vi "UART_With_Buffer.vi"(0 "COM":refnum<visa-resource-name>, 1 "Send":string(combo), 3 "Timeout (ms)":u32=500, 5 "Function":T1(ring)=enum."SendWaitRead", 9 "Baudrate":u32=3000000, 11 "error in (no error)":errorcluster, 12 "REC":string) -> (4 "ReceiveString":string, 6 "pass?":bool, 10 "Return":string, 15 "error out":errorcluster)   [LabVIEW 2020, in "UART.lvlib"]
uses:
  UART.lvlib
  <vilib>/Instr/_visa.llb/VISA Set IO Buffer Mask.ctl
  <vilib>/Instr/_visa.llb/VISA Flush IO Buffer Mask.ctl
  4a145ab3-8364-4eaa-b6a3-0a612f5f0f50.vi
  75df8ced-9b69-4a5e-8517-458ef4cbff5d.vi
  <vilib>/Instr/_visa.llb/VISA Configure Serial Port (Instr).vi
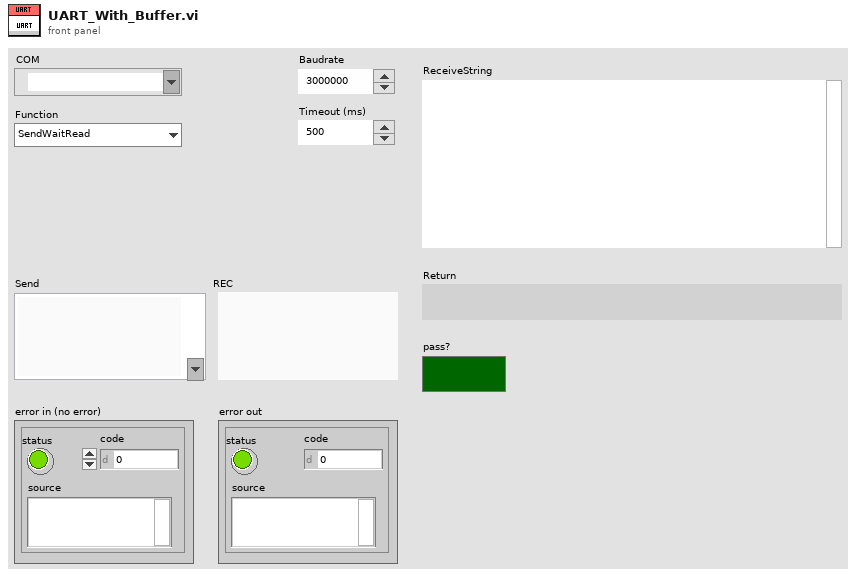
[diagram p1: front panel]
types:
  T1 = enum16{"Open", "Close", "ClearBuffer", "Send", "Read", "SendWaitRead", "SendCompare", "ReadCompare"}
  T2 = typedef "VISA Set IO Buffer Mask.ctl" = u16
  T3 = typedef "VISA Flush IO Buffer Mask.ctl" = u16
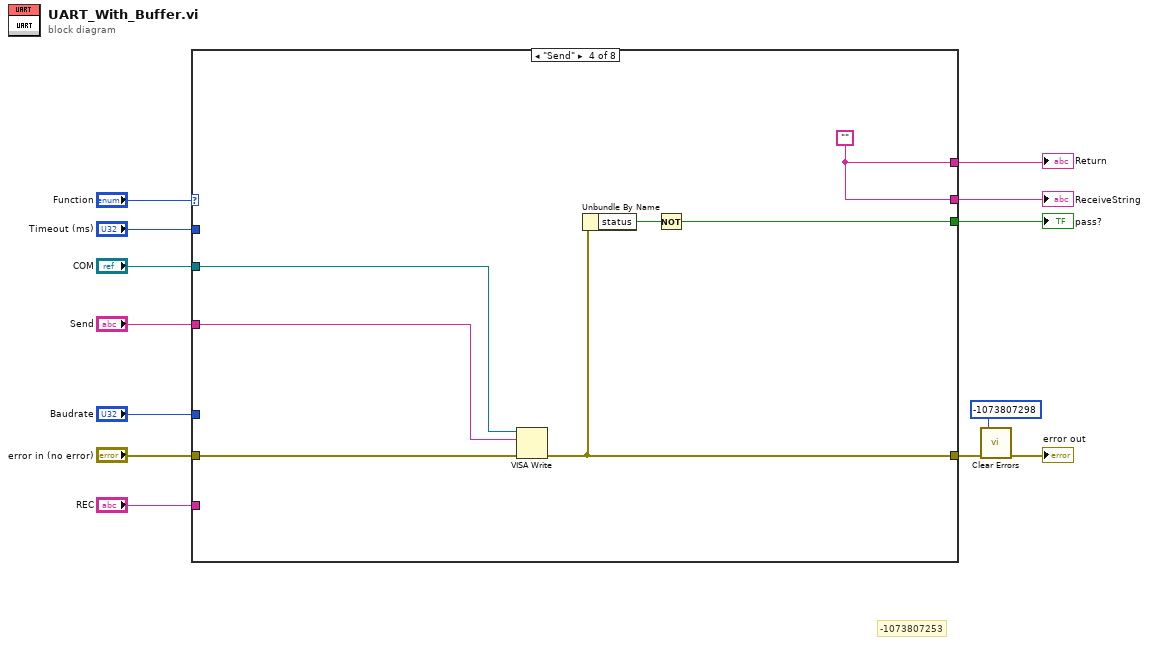
[diagram p0: block diagram]
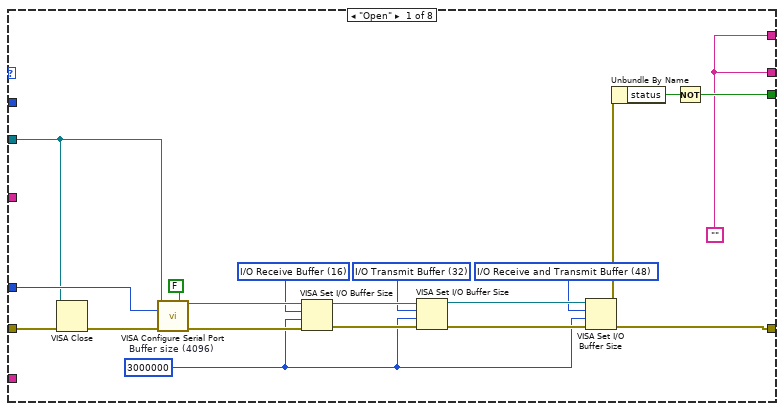
[diagram p2: hidden frame]
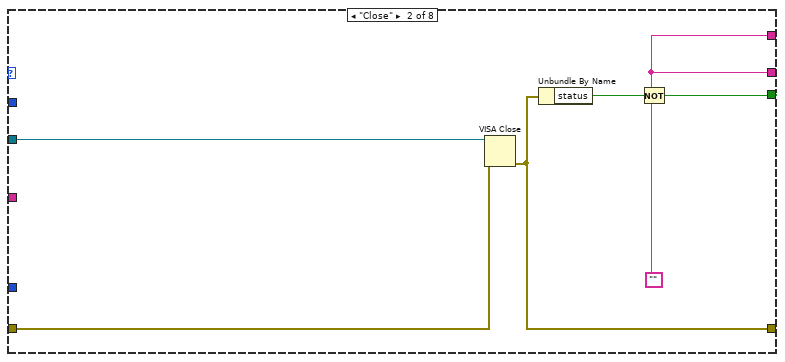
[diagram p3: hidden frame]
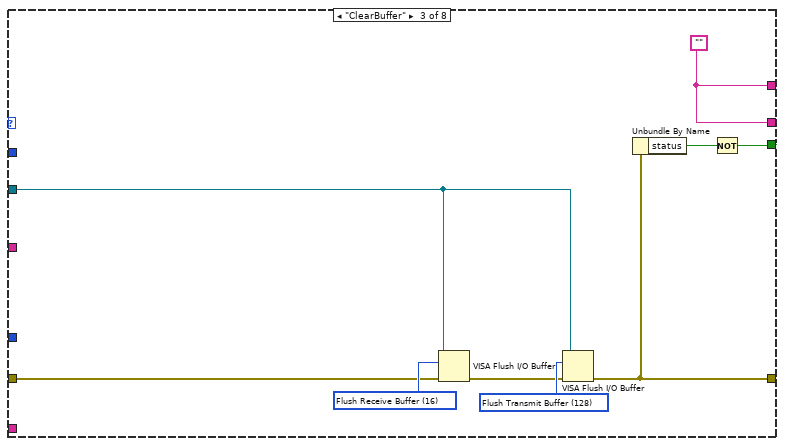
[diagram p4: hidden frame]
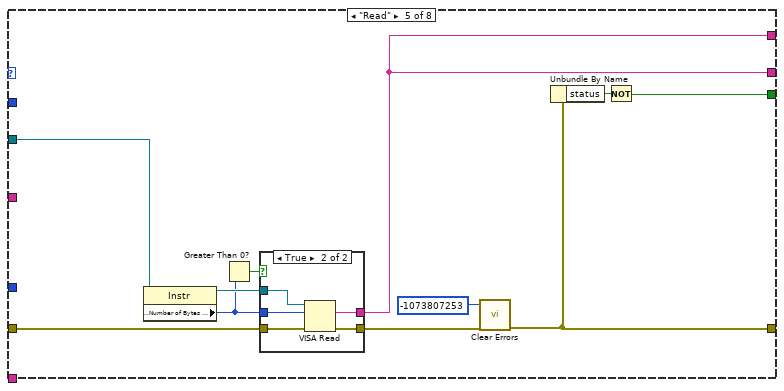
[diagram p5: hidden frame]
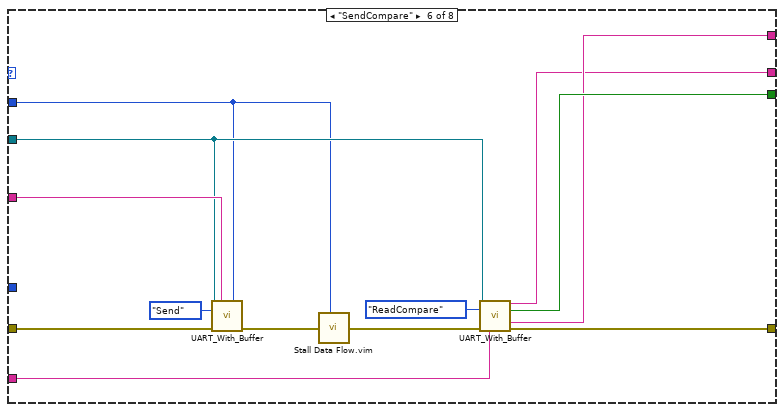
[diagram p7: hidden frame]
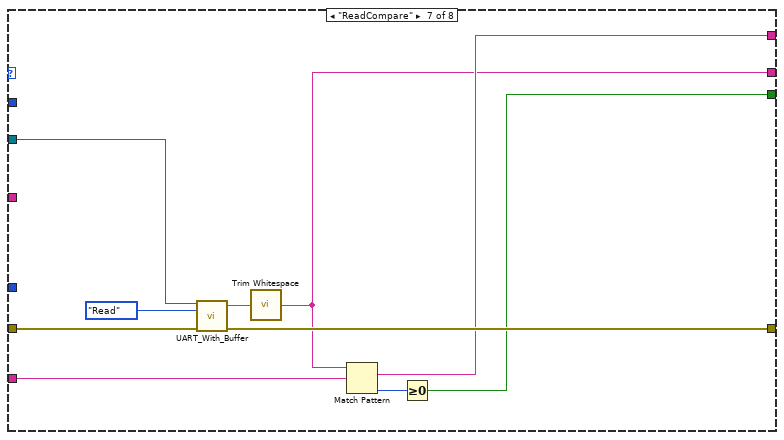
[diagram p8: hidden frame]
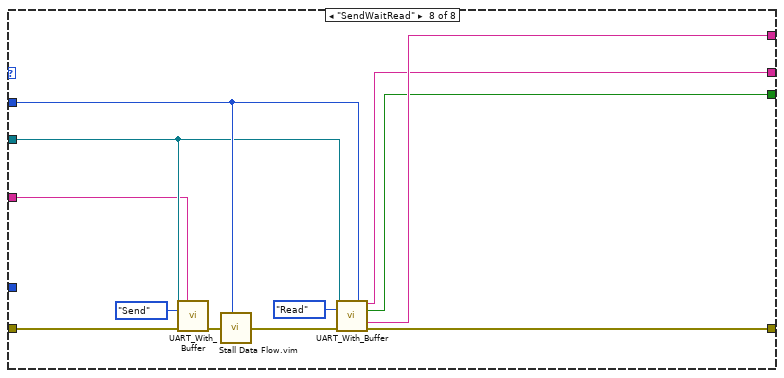
[diagram p9: hidden frame]
diagram:
  # "-1073807253"
  n1 = case shown="\"Send\"" "Function" {
    tunnel: "Send" -> [_ _ _ w49 _ w84 _ w100]
    tunnel: "error in (no error)" -> [w28 w35 w40 w52 w63 w80 w93 w99]
    tunnel: [w15 w34 w43 w53 w55 w83 w92 w106] -> w4
    tunnel: [w32 w37 w46 w48 w58 w82 w91 w104] -> w13
    tunnel: "COM" -> [w29 w36 w39 w51 w64 w78 w94 w101]
    tunnel: "Baudrate" -> [w31 _ _ _ _ _ _ _]
    tunnel: "Timeout (ms)" -> [_ _ _ _ _ w74 _ w102]
    tunnel: "REC" -> [_ _ _ _ _ w77 w86 _]
    tunnel: [w14 w33 w45 w50 w59 w81 w90 w105] -> w2
    tunnel: [w14 w33 w45 w50 w59 w76 w87 w97] -> w1
    frame "Open" {
      w17 = T2 16 items=["I/O Receive Buffer"=16, "I/O Transmit Buffer"=32, "I/O Receive and Transmit Buffer"=48] ("Mask")
      w18 = T2 48 items=["I/O Receive Buffer"=16, "I/O Transmit Buffer"=32, "I/O Receive and Transmit Buffer"=48] ("Mask")
      w19 = T2 32 items=["I/O Receive Buffer"=16, "I/O Transmit Buffer"=32, "I/O Receive and Transmit Buffer"=48] ("Mask")
      w20 = u32 3000000  # Buffer size (4096)
      w14 = ""
      n2 = VISA Close(VISA resource name=w29, error in (no error)=w28) -> (error out=w27:errorcluster)
      n3 = call-poly "VISA Configure Serial Port"("VISA resource name"=w29, "Enable Termination\nChar (T)"=FALSE ("Enable Termination\nChar (T)"), "baud rate (9600)"=w31, "error in (no error)"=w27) -> ("VISA resource name out"=w25:refnum<visa-resource-name>, "error out"=w26:errorcluster)  [unwired: 4 in, 6 out]
      n4 = VISA Set I/O Buffer Size(VISA resource name=w25, mask (16)=w17, size (4096)=w20, error in (no error)=w26) -> (VISA resource name out=w24:refnum<visa-resource-name>, error out=w22:errorcluster)
      n5 = VISA Set I/O Buffer Size(VISA resource name=w24, mask (16)=w19, size (4096)=w20, error in (no error)=w22) -> (VISA resource name out=w23:refnum<visa-resource-name>, error out=w21:errorcluster)
      n6 = VISA Set I/O Buffer Size(VISA resource name=w23, mask (16)=w18, size (4096)=w20, error in (no error)=w21) -> (error out=w15:errorcluster)  [unwired: 1 out]
      n7 = Unbundle By Name(w15) -> ("status"=w16:bool)
      n8 = Not(x=w16) -> (.not. x?=w32:bool)
    }
    frame "Close" {
      w33 = ""
      n9 = VISA Close(VISA resource name=w36, error in (no error)=w35) -> (error out=w34:errorcluster)
      n10 = Unbundle By Name(w34) -> ("status"=w38:bool)
      n11 = Not(x=w38) -> (.not. x?=w37:bool)
    }
    frame "ClearBuffer" {
      w42 = T3 16 items=["Flush Receive Buffer"=16, "Write Transmit Buffer to Device"=32, "Flush Receive Buffer (No I/O)"=64, "Flush Transmit Buffer"=128] ("Mask")
      w44 = T3 128 items=["Flush Receive Buffer"=16, "Write Transmit Buffer to Device"=32, "Flush Receive Buffer (No I/O)"=64, "Flush Transmit Buffer"=128] ("Mask")
      w45 = ""
      n12 = VISA Flush I/O Buffer(VISA resource name=w39, mask (16)=w42, error in (no error)=w40) -> (error out=w41:errorcluster)  [unwired: 1 out]
      n13 = VISA Flush I/O Buffer(VISA resource name=w39, mask (16)=w44, error in (no error)=w41) -> (error out=w43:errorcluster)  [unwired: 1 out]
      n14 = Unbundle By Name(w43) -> ("status"=w47:bool)
      n15 = Not(x=w47) -> (.not. x?=w46:bool)
    }
    frame "Send" {
      w50 = ""
      n16 = VISA Write(VISA resource name=w51, write buffer=w49, error in (no error)=w52) -> (error out=w53:errorcluster)  [unwired: 2 out]
      n17 = Unbundle By Name(w53) -> ("status"=w54:bool)
      n18 = Not(x=w54) -> (.not. x?=w48:bool)
    }
    frame "Read" {
      n19 = property class="Instr"(reference=w64) -> (reference out=w62:refnum<visa-resource-name>, "Serial Settings:Number of Bytes at Serial Port"=w61:u32)  [unwired: 1 in, 1 out]
      n20 = Greater Than 0?(x=w61) -> (x > 0?=w60:bool)
      n21 = case shown="True" w60 {
        tunnel: [w66 w71] -> w56
        tunnel: w63 -> [w66 w70]
        tunnel: w62 -> [_ w69]
        tunnel: [_ w68] -> w59
        tunnel: w61 -> [_ w67]
        frame False {
        }
        frame True {
          n22 = VISA Read(VISA resource name=w69, byte count=w67, error in (no error)=w70) -> (read buffer=w68:string, error out=w71:errorcluster)  [unwired: 2 out]
        }
      }
      n23 = call <vilib>:"Clear Errors.vi"("error in (no error)"=w56, "specific error code to clear (0: all)"=-1073807253) -> ("error out"=w55:errorcluster)  [unwired: 4 in, 1 out]
      n24 = Unbundle By Name(w55) -> ("status"=w65:bool)
      n25 = Not(x=w65) -> (.not. x?=w58:bool)
    }
    frame "SendCompare" {
      n26 = call "UART_With_Buffer.vi"("COM"=w78, "Send"=w84, "Timeout (ms)"=w74, "Function"=T1."Send", "error in (no error)"=w80) -> ("error out"=w79:errorcluster)  [unwired: 7 in, 3 out]
      n27 = call "Stall Data Flow.vim"("value in"=w79, "milliseconds to wait"=w74) -> ("value out"=w75:errorcluster)  [unwired: 1 out]
      n28 = call "UART_With_Buffer.vi"("COM"=w78, "Function"=T1."ReadCompare", "error in (no error)"=w75, "REC"=w77) -> ("ReceiveString"=w76:string, "pass?"=w82:bool, "Return"=w81:string, "error out"=w83:errorcluster)  [unwired: 8 in]
    }
    frame "ReadCompare" {
      n29 = call "UART_With_Buffer.vi"("COM"=w94, "Function"=T1."Read", "error in (no error)"=w93) -> ("ReceiveString"=w88:string, "error out"=w92:errorcluster)  [unwired: 9 in, 2 out]
      n30 = call <vilib>:"Trim Whitespace.vi"("string"=w88) -> ("trimmed string"=w87:string)  [unwired: 1 in]
      n31 = Match Pattern(string=w87, regular expression=w86) -> (match substring=w90:string, offset past match=w89:i32)  [unwired: 1 in, 2 out]
      n32 = Greater Or Equal To 0?(x=w89) -> (x >= 0?=w91:bool)
    }
    frame "SendWaitRead" {
      n33 = call "UART_With_Buffer.vi"("COM"=w101, "Send"=w100, "Function"=T1."Send", "error in (no error)"=w99) -> ("error out"=w98:errorcluster)  [unwired: 8 in, 3 out]
      n34 = call "Stall Data Flow.vim"("value in"=w98, "milliseconds to wait"=w102) -> ("value out"=w103:errorcluster)  [unwired: 1 out]
      n35 = call "UART_With_Buffer.vi"("COM"=w101, "Timeout (ms)"=w102, "Function"=T1."Read", "error in (no error)"=w103) -> ("ReceiveString"=w97:string, "pass?"=w104:bool, "Return"=w105:string, "error out"=w106:errorcluster)  [unwired: 8 in]
    }
  }
  "pass?" <- w13
  "Return" <- w2
  "ReceiveString" <- w1
  n36 = call <vilib>:"Clear Errors.vi"("error in (no error)"=w4, "specific error code to clear (0: all)"=-1073807298) -> ("error out"=→"error out":errorcluster)  [unwired: 4 in, 1 out]
